vi "CsTool-InitializeFill.vi"() -> (0 "Error Code":i32, 1 "Number Of Systems":i32)   [LabVIEW 2022 SP3]
doc: "This VI initializes the CompuScope driver and returns the total number of CompuScope systems. \n\nIf the call is successful, the Error Code will show the number of systems. If the call is unsuccessful, the Number Of Systems is returned as 0 and an appropriate error code is returned in the Error Code indicator. A descriptive error string may be obtained by calling CsTool-ErrorHandler.vi."
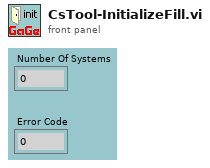
[diagram p1: front panel]
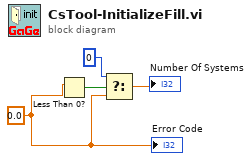
[diagram p0: block diagram]
diagram:
  w1 = 0.0 ("x")
  n1 = Less Than 0?(x=w1) -> (x < 0?=w4:bool)
  n2 = Select(t=0, s=w4, f=w1) -> (s? t:f=→"Number Of Systems":dbl)
  "Error Code" <- w1
